vi "PFMate-DM.vi"(0 "Inputs":T1={"Dir A"=TRUE, "MA"=0, "MB"=0, "Operation"=0, "Pwr A"=5, "Pwr B"=5, "Dir B"=TRUE, "Channel"=1, "PFMate address 2"=72} {"PFMate address 2" format="%x"; "Pwr B" min=1 max=7 step=1 scale=1.0..7.0; "Pwr A" min=1 max=7 step=1 scale=1.0..7.0; "MB" items=["Run", "Float", "Brake"]; "MA" items=["Run", "Float", "Brake"]}, 2 "NXT":T3={"Hardware"="NXT", "Flattened String"=""}, 3 "Input Port":T2 items=["Port 1", "Port 2", "Port 3", "Port 4"]) -> (4 "NXT dup":T3={"Hardware"="NXT", "Flattened String"=""})   [LabVIEW 2011]
uses:
  <vilib>/NXT/Subs/LVHSConnector.ctl
  <vilib>/NXT/Block Support/NXT_InputPort.ctl
  <vilib>/NXT/Block Support/HWPage.SensorType.ctl
  <vilib>/NXT/Block Support/HWPage.SensorMode.ctl
panel:
  out "Operation":u8
  # "mindsensors.com\nCopyright (c) 2009 by mindsensors.com\nEmail: info (<at>) mindsensors (<dot>) com\n\nThis program is free software. You can redistribute it and/or modify\nit under the terms of the GNU General Public License as published by\nthe Free Software Foundation; version 3 of the License.\nRead the license at: http://www.gnu.org/licenses/gpl.txt"
  # "Motor A"
  # "Motor B"
  # "Mode"
  # "Direction"
  # "Power"
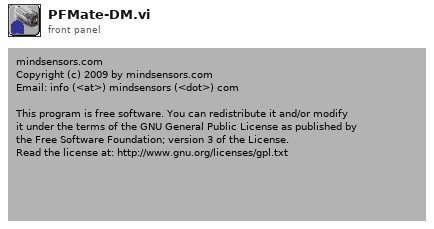
[diagram p1: front panel]
types:
  T1 = cluster{"Dir A":bool, "MA":u8, "MB":u8, "Operation":u8, "Pwr A":u8, "Pwr B":u8, "Dir B":bool, "Channel":u8, "PFMate address 2":u8}
  T2 = typedef "NXT_InputPort.ctl" = u8
  T3 = typedef "LVHSConnector.ctl" = cluster{"Hardware":string, "Flattened String":string}
  T4 = typedef "HWPage.SensorType.ctl" = u8
  T5 = typedef "HWPage.SensorMode.ctl" = u8
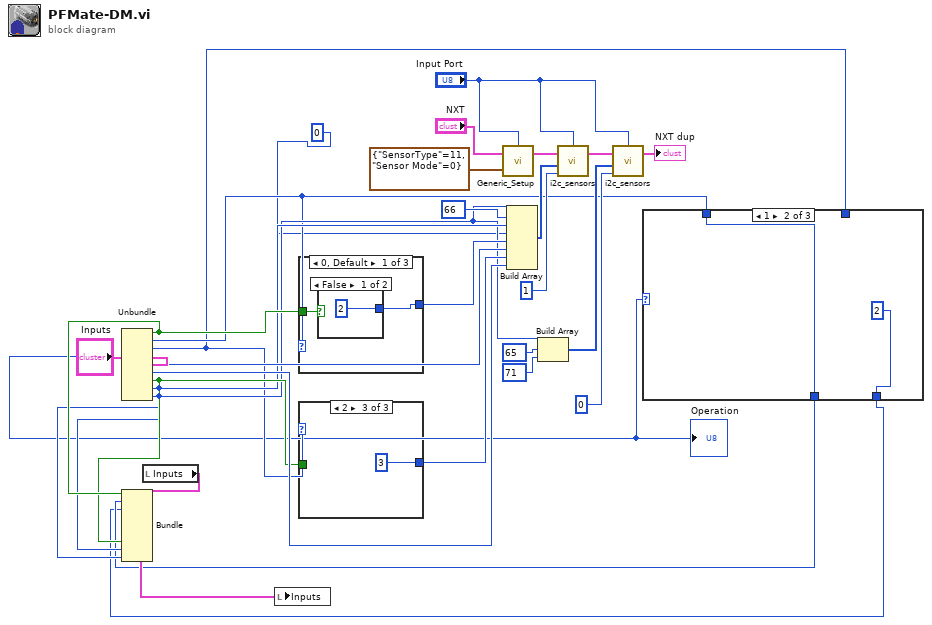
[diagram p0: block diagram]
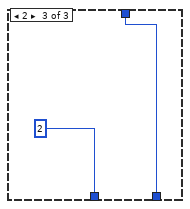
[diagram p3: hidden frame]
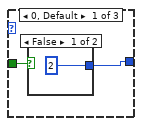
[diagram p4: hidden frame]
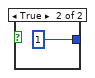
[diagram p5: hidden frame]
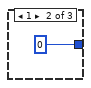
[diagram p6: hidden frame]
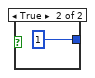
[diagram p7: hidden frame]
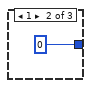
[diagram p8: hidden frame]
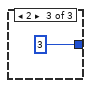
[diagram p9: hidden frame]
diagram:
  n1 = Unbundle("Inputs") -> ("Dir A"=w10:bool, "MA"=w4:u8, "MB"=w3:u8, "Operation"=w2:u8, "Pwr A"=w25:u8, "Pwr B"=w24:u8, "Dir B"=w9:bool, "Channel"=w8:u8, "PFMate address 2"=w7:u8)
  "Operation" <- w2
  n2 = local read "Inputs"() -> (w11:T1)
  n3 = case shown="0, Default" w4 {
    tunnel: w10 -> [w32 _ _]
    tunnel: [w31 0 3] -> w29
    frame 0, Default {
      n4 = case shown="False" w32 {
        tunnel: [2 1] -> w31
        frame False {
        }
        frame True {
        }
      }
    }
    frame 1 {
    }
    frame 2 {
    }
  }
  n5 = case shown="2" w3 {
    tunnel: w9 -> [w38 _ _]
    tunnel: [w37 0 3] -> w28
    frame 0, Default {
      n6 = case shown="False" w38 {
        tunnel: [2 1] -> w37
        frame False {
        }
        frame True {
        }
      }
    }
    frame 1 {
    }
    frame 2 {
    }
  }
  n7 = call <vilib>:"Generic_Setup.vi"("Sensor Setup"=cluster{"SensorType":T4, "Sensor Mode":T5} {"SensorType"=11, "Sensor Mode"=0}, "NXT"="NXT", "Port"="Input Port") -> ("NXT"=w18:T3)  [unwired: 1 out]
  n8 = Build Array(w7, u8 66 ("register"), w8, 0, w29, w25, w28, w24) -> (w14:i32[])
  n9 = Build Array(w7, u8 65 ("register"), u8 71 ("register")) -> (w21:u8[])
  n10 = call <vilib>:"i2c_sensors.vi"("Return Length"=u8 1, "Bytes to Write"=w14, "NXT"=w18, "Port"="Input Port") -> ("NXT"=w17:T3)  [unwired: 1 in, 2 out]
  n11 = call <vilib>:"i2c_sensors.vi"("Return Length"=u8 0, "Bytes to Write"=w21, "NXT"=w17, "Port"="Input Port") -> ("NXT"=→"NXT dup":T3)  [unwired: 1 in, 2 out]
  n12 = case shown="1" w2 {
    tunnel: [w44 w46 2] -> w6
    tunnel: [w43 2 w48] -> w5
    tunnel: w4 -> [w44 w46 _]
    tunnel: w3 -> [w43 _ w48]
    frame 0, Default {
    }
    frame 1 {
    }
    frame 2 {
    }
  }
  n13 = Bundle(cluster=w11, "Dir A"=w10, "MA"=w6, "MB"=w5, "Dir B"=w9, "Channel"=w8, "PFMate address 2"=w7) -> (w12:T1)  [unwired: 3 in]
  n14 = local write "Inputs"(w12) -> ()
